vi "PPT Server.vi"(11 "DVR In":refnum<data-value>) -> (3 "DVR Out":refnum<data-value>)   [LabVIEW 2015]
uses:
  Data/Nicholas Data.lvclass
  Devices/PPT/PPT.lvclass
  Session/Raw FPGA/FPGA Session.lvclass
  Reusable/Session Log/System Log.lvclass
  Reusable/Session APIs/File Access/Config Data/Config Data.lvclass
  Session/FPGA Serial Session.lvclass
  Reusable/Session APIs/File Access/Config Data/Config Data.lvclass/Config Data.ctl
  Reusable/Session Log/System Log.lvclass/System Log.ctl
  <vilib>/Platform/TimedLoop/XDataNode/timing_clust.ctl
  <vilib>/Platform/TimedLoop/XDataNode/nitl_modes.ctl
  <vilib>/Platform/TimedLoop/XDataNode/wakeup.ctl
  Devices/PPT/PPT.lvclass/PPT.ctl
  Session/FPGA Serial Session.lvclass/FPGA Serial Session.ctl
  Reusable/Session APIs/Text Communication/Text Device Session.lvclass/Text Device Session.ctl
  Devices/Configurable Device/Configurable Device.lvclass/Configurable Device.ctl
  Reusable/Data/Array Data/Single 1-D/Single_Array.lvclass
  Data/Nicholas Data.lvclass/Nicholas Data.ctl
  Devices/PPT/Accessors/Write ID.vi
  Session/Write fpgaSession.vi
  Reusable/Session APIs/Text Communication/Write hSysLog.vi
  Devices/Configurable Device/Write Handle.vi
  Devices/PPT/Accessors/Write hSession.vi
  Data/Write PPT Data.vi
  Reusable/Session APIs/File Access/Config Data/Accessors/Write Cfg Path.vi
  Reusable/Session Log/Accessors/Write Main Path.vi
  <vilib>/Platform/TimedLoop/XDataNode/XDataNode.xnode
  <userlib>/_Session Fwk/Session - Root.lvclass
  <vilib>/Platform/TimedLoop/XDataNode/XDNodeRunTimeDep.lvlib
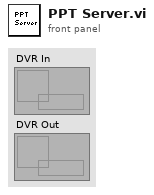
[diagram p1: front panel]
types:
  T1 = typedef "Session - Root.lvclass/Session Handle.ctl" = refnum<data-value>
  T2 = typedef "XDNodeRunTimeDep.lvlib/timing_clust.ctl" = cluster{"Expected End [f-1]":u64, "Actual End [f-1]":u64, "Finished Late? [f-1]":bool, "Expected End [i-1]":u64, "Actual End [i-1]":u64, "Finished Late? [i-1]":bool, "Expected Start [i]":u64, "Actual Start [i]":u64, "Expected Start [f]":u64, "Actual Start [f]":u64, "Source Name":string, "Structure Name":string, "Period":i64, "Deadline":i64, "Offset":i64, "Start":i64, "Priority":i32, "Timeout":i32, "Mode":T3, "Wakeup Reason":T4, "Error":errorcluster, "Source Type":string, "Secondary Source Type":string, "Global End Time":u64, "Global Start Time":u64, "Frame Duration":u64, "Iteration Duration":u64, "Assigned CPU":i32, "I/O Scan Engine Mode":u32}
  T3 = typedef "XDNodeRunTimeDep.lvlib/nitl_modes.ctl" = enum32{"No Change", "Process missed periods, maintain original phase", "Discard missed periods, maintain original phase", "Process missed periods, ignore original phase", "Discard missed periods, ignore original phase"}
  T4 = typedef "XDNodeRunTimeDep.lvlib/wakeup.ctl" = enum32{"Normal", "Aborted", "Asynchronous wakeup", "Timing source error", "Timed loop error", "Timeout"}
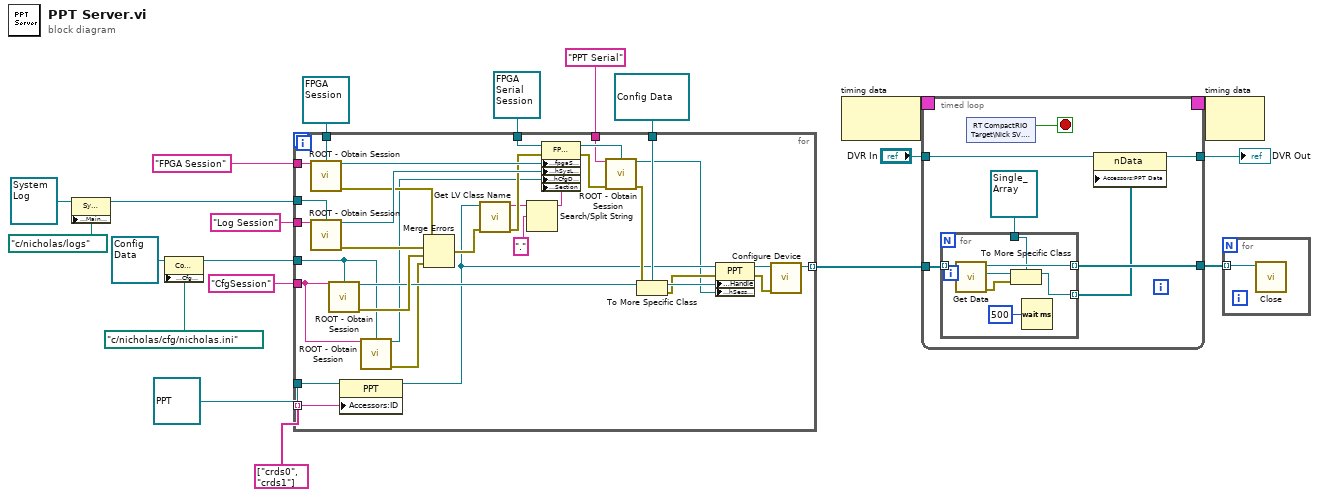
[diagram p0: block diagram]
diagram:
  n1 = property class="Sys Log"(reference=refnum<class "System Log.lvclass"> refnum ("Sys Log"), "Accessors:Main Path"=path "c:/nicholas/logs" ("Main Path")) -> (reference out=w10:refnum<class "System Log.lvclass">)  [unwired: 1 in, 1 out]
  n2 = property class="Config Data"(reference=refnum<class "Config Data.lvclass"> refnum ("Config Data"), "Accessors:Cfg Path"=path "c:/nicholas/cfg/nicholas.ini" ("Cfg Path")) -> (reference out=w11:refnum<class "Config Data.lvclass">)  [unwired: 1 in, 1 out]
  n3 = for {
    tunnel: w10 -> [w55]
    tunnel: "Log Session" ("Session Name ()") -> [w54]
    tunnel: refnum<class "FPGA Session.lvclass"> refnum ("FPGA Session") -> [w53]
    tunnel: "FPGA Session" ("Session Name ()") -> [w52]
    tunnel: w11 -> [w31]
    tunnel: "CfgSession" ("Session Name ()") -> [w32]
    tunnel: refnum<class "FPGA Serial Session.lvclass"> refnum ("FPGA Serial Session.lvclass") -> [w50]
    tunnel: refnum<data-value> refnum ("Session Handle") -> [w39]
    tunnel: "PPT Serial" ("Session Name ()") -> [w33]
    tunnel: string[] ["crds0", "crds1"] -> [w28] mode=indexing
    tunnel: refnum<class "PPT.lvclass"> refnum ("PPT") -> [w27]
    tunnel: [w22] -> w5 mode=indexing
    n4 = call <userlib>:"ROOT - Obtain Session.vi"("Session Name ()"=w52, "OBJ - Session"=w53) -> ("Session Handle"=w51:T1, "error out"=w47:errorcluster)  [unwired: 11 in, 1 out]
    n5 = call <userlib>:"ROOT - Obtain Session.vi"("Session Name ()"=w54, "OBJ - Session"=w55) -> ("Session Handle"=w48:T1, "error out"=w46:errorcluster)  [unwired: 11 in, 1 out]
    n6 = call <userlib>:"ROOT - Obtain Session.vi"("Session Name ()"=w32, "OBJ - Session"=w31) -> ("Session Handle"=w43:T1, "error out"=w45:errorcluster)  [unwired: 11 in, 1 out]
    n7 = property class="PPT"(reference=w27, "Accessors:ID"=w28) -> (reference out=w26:refnum<class "PPT.lvclass">)  [unwired: 1 in, 1 out]
    n8 = call <userlib>:"ROOT - Obtain Session.vi"("Session Name ()"=w32, "OBJ - Session"=w31) -> ("Session Handle"=w30:T1, "error out"=w29:errorcluster)  [unwired: 11 in, 1 out]
    n9 = Merge Errors(w47, w46, w45, w29) -> (w38:errorcluster)
    n10 = call <vilib>:"Get LV Class Name.vi"("error in (no error)"=w38, "object"=w26) -> ("error out"=w37:errorcluster, "class name"=w35:string)  [unwired: 8 in]
    n11 = Search/Split String(string=w35, search string/char (-)="." ("regular expression")) -> (substring before match=w34:string)  [unwired: 1 in, 2 out]
    n12 = property class="FPGA Serial Session"(reference=w50, error in=w37, "Accessors:fpgaSession"=w51, "Accessors:hSysLog"=w48, "Accessors:hCfgData"=w30, "Accessors:Section"=w34) -> (reference out=w49:refnum<class "FPGA Serial Session.lvclass">, error out=w44:errorcluster)
    n13 = call <userlib>:"ROOT - Obtain Session.vi"("Session Name ()"=w33, "OBJ - Session"=w49, "error in (no error)"=w44) -> ("Session Handle"=w25:T1, "error out"=w41:errorcluster)  [unwired: 10 in, 1 out]
    n14 = To More Specific Class(target class=w39, reference=w43, error in=w41) -> (specific class reference=w42:refnum<data-value>, error out=w40:errorcluster)
    n15 = property class="PPT"(reference=w26, error in=w40, "Accessors:Handle"=w42, "Accessors:hSession"=w25) -> (reference out=w24:refnum<class "PPT.lvclass">, error out=w23:errorcluster)
    n16 = call-dynamic "Configure Device.vi"("error in"=w23, "PPT in"=w24) -> ("PPT out"=w22:refnum<class "PPT.lvclass">)  [unwired: 8 in, 1 out]
  }
  n17 = node-c288() -> (w7:T2)  [unwired: 1 in]
  n18 = timed-loop {
    tunnel: w5 -> [w62]
    tunnel: [w61] -> w1
    timing: w7 -> [_]
    timing-out: [_] -> w6
    tunnel: "DVR In" -> [w59]
    tunnel: [w57] -> w3
    stop <- w60 stop-if-true
    n19 = for {
      tunnel: w62 -> [w69] mode=indexing
      tunnel: [w68] -> w61 mode=indexing
      tunnel: refnum<class "Single_Array.lvclass"> refnum ("Base Data Lib:[SGL]") -> [w66]
      tunnel: [w65] -> w56 mode=indexing
      n20 = call-dynamic "Get Data.vi"("Cfg Dev in"=w69) -> ("error out"=w64:errorcluster, "Data"=w67:refnum<class "Data.lvclass">, "Cfg Dev out"=w68:refnum<class "PPT.lvclass">)  [unwired: 8 in]
      n21 = To More Specific Class(target class=w66, reference=w67, error in=w64) -> (specific class reference=w65:refnum<class "Single_Array.lvclass">)  [unwired: 1 out]
      n22 = Wait (ms)(milliseconds to wait=u32 500) -> ()  [unwired: 1 out]
    }
    n23 = shared-variable "RT CompactRIO Target\\Nick SV.lvlib\\Stop"() -> (w60:bool)  [unwired: 1 in, 1 out]
    n24 = property class="nData"(reference=w59, "Accessors:PPT Data"=w56) -> (reference out=w57:refnum<data-value>)  [unwired: 1 in, 1 out]
  }
  "DVR Out" <- w3
  n25 = node-c288(w6) -> ()  [unwired: 1 out]
  n26 = for {
    tunnel: w1 -> [w72] mode=indexing
    n27 = call-dynamic "Close.vi"("Cfg Dev in"=w72) -> ()  [unwired: 9 in, 2 out]
  }
